vi "Split.vi"(6 "Groups":string[][](array[string]), 8 "error in (no error)":errorcluster caption="entrée d'erreur (pas d'erreur)", 9 "y":string[][](array[string]), 10 "X":string[][](array[string]), 11 "ShuffleSplit.lvclass":refnum<class "ShuffleSplit.lvclass">) -> (0 "error out":errorcluster caption="sortie d'erreur", 2 "Split":T1(array[cluster]), 3 "ShuffleSplit.lvclass":refnum<class "ShuffleSplit.lvclass">)   [LabVIEW 2020, in "ShuffleSplit.lvclass"]
doc: "Returns :\n- train : ndarray\n The training set indices for that split.\n\n- test : ndarray\n The testing set indices for that split."
uses:
  ShuffleSplit.lvclass
  ShuffleSplit.lvclass/ShuffleSplit.ctl
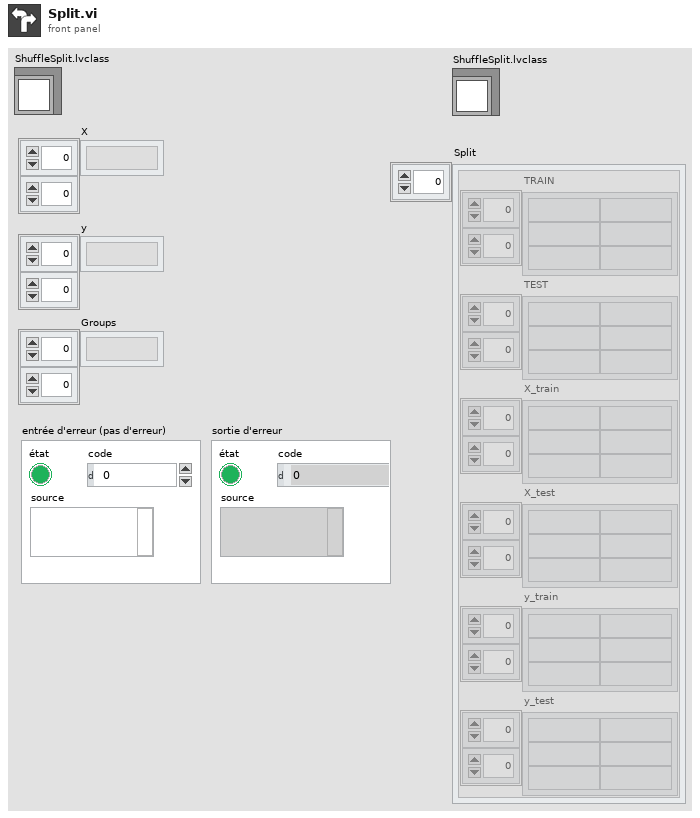
[diagram p1: front panel]
types:
  T1 = cluster{"TRAIN":string[][], "TEST":string[][], "X_train":string[][], "X_test":string[][], "y_train":string[][], "y_test":string[][]}[]
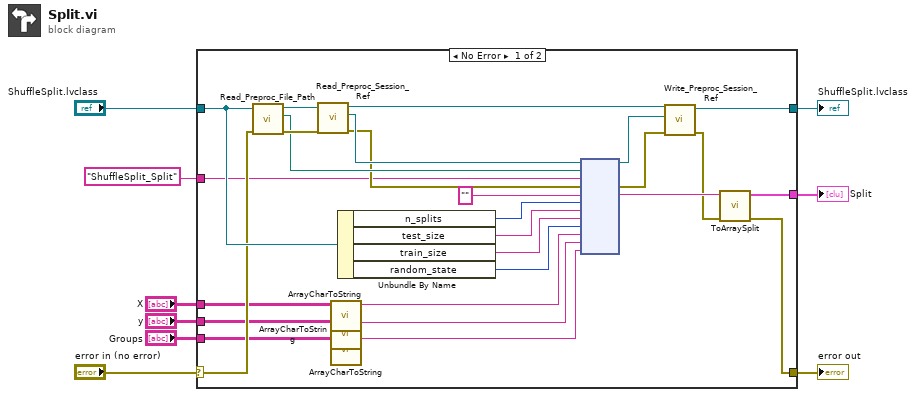
[diagram p0: block diagram]
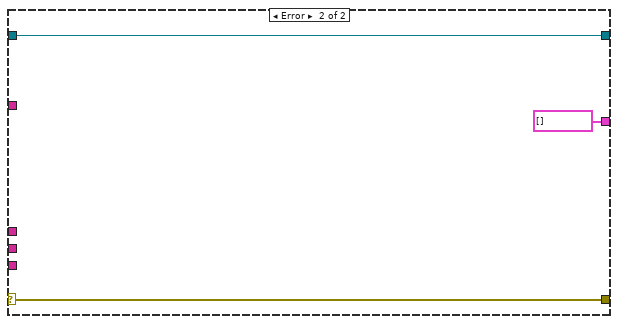
[diagram p2: hidden frame]
diagram:
  n1 = case shown="No Error" "error in (no error)" {
    selector: "error in (no error)" -> [w26 w39]
    tunnel: [w11 w39] -> w8
    tunnel: [w13 w38] -> w6
    tunnel: "ShuffleSplit.lvclass" -> [w27 w38]
    tunnel: "ShuffleSplit_Split" -> [w25 _]
    tunnel: "X" -> [w20 _]
    tunnel: "y" -> [w19 _]
    tunnel: "Groups" -> [w18 _]
    tunnel: [w10 T1 [] ("Split")] -> w1
    frame No Error {
      n2 = call-dynamic "Read_Preproc_File_Path.vi"("error in (no error)"=w26, "Python in"=w27) -> ("error out"=w35:errorcluster, "File_Path"=w34:path, "Python out"=w36:refnum<class "ShuffleSplit.lvclass">)  [unwired: 7 in]
      n3 = call-dynamic "Read_Preproc_Session_Ref.vi"("error in (no error)"=w35, "Python in"=w36) -> ("error out"=w32:errorcluster, "Session_ref"=w33:refnum<k35>, "Python out"=w31:refnum<class "ShuffleSplit.lvclass">)  [unwired: 7 in]
      n4 = call "ArrayCharToString.vi"("TAB"=w20) -> ("Instruction"=w17:string)  [unwired: 10 in]
      n5 = call "ArrayCharToString.vi"("TAB"=w19) -> ("Instruction"=w16:string)  [unwired: 10 in]
      n6 = call "ArrayCharToString.vi"("TAB"=w18) -> ("Instruction"=w15:string)  [unwired: 10 in]
      n7 = Unbundle By Name(w27) -> ("n_splits"=w24:i32, "test_size"=w23:string, "train_size"=w22:string, "random_state"=w21:i32)
      n8 = node(w33, w34, w25, w32, "", w24, w23, w22, w21, w17, w16, w15) -> (w29:refnum<k35>, w30:errorcluster, w14:string)  [unwired: 7 in, 2 out]
      n9 = call-dynamic "Write_Preproc_Session_Ref.vi"("error in (no error)"=w30, "Session_ref"=w29, "Python in"=w31) -> ("error out"=w12:errorcluster, "Python out"=w13:refnum<class "ShuffleSplit.lvclass">)  [unwired: 7 in]
      n10 = call "ToArraySplit.vi"("sortie d'erreur"=w12, "Return value"=w14) -> ("sortie d'erreur"=w11:errorcluster, "Split"=w10:T1)  [unwired: 8 in]
    }
    frame Error {
    }
  }
  "error out" <- w8
  "ShuffleSplit.lvclass" <- w6
  "Split" <- w1
